vi "Tração cond a AT  subvão.vi"(8 "error in (no error)":errorcluster, 11 "Dados SP":T1={"Condutor"={"Pc (N/m)"=0.0, "Mod.Young (N/m²)"=0.0, "Dil.Term.c (m/°C)"=0.0, "Área  (m²)"=0.0, "Tração EDS (N)"=0.0, "Tração Torig(N)"=0.0, "Tração Talta (N)"=0.0}, "Suporte"={"Ps (N/m)"=0.0, "Es (N/m²)"=0.0, "DTc (1/°C)"=0.0, "Área sup (m²)"=0.0, "Tração EDS sup (N)"=0.0, "Tração AT sup (N)"=0.0, "Flecha sup AT (m)"=0.0}, "Projeto"={"Temp. EDS (°C)"=0.0, "Lim.original (°C)"=0.0, "Lim.extend. (°C)"=0.0, "N. cabo/fase"=1.0}, "Vetor de dados"={"Coor.X.esp"=[], "Coor.Y.Esp."=[], "Sub.vao X"=[], "Sub.vao Y"=[], "CoordY.sup"=[], "CoordX.sup"=[]}, "Subvão"={"N. Esp."=0.0, "F.lim (m)"=0.0, "Ext.calc"=0.0, "Ext.definido"=0.0, "Comp.cabo"=0.0, "Ext.55%"=0.0, "Tração sub\nAT (N)"=0.0, "Ext.sel."=0.0, "Flecha lim.\ncalc (m)"=0.0}, "Vão"={"Extensão (m)"=0.0, "Desnivel (m)"=0.0, "Ext.Lim sub (m)"=0.0, "Flecha à 60 °C"=0.0}} {"Projeto"."N. cabo/fase" min=1.0 max=8.0 step=1.0 format="%#_1f"}) -> (0 "error out":errorcluster, 3 "Dados SP Out":T1={"Condutor"={"Pc (N/m)"=0.0, "Mod.Young (N/m²)"=0.0, "Dil.Term.c (m/°C)"=0.0, "Área  (m²)"=0.0, "Tração EDS (N)"=0.0, "Tração Torig(N)"=0.0, "Tração Talta (N)"=0.0}, "Suporte"={"Ps (N/m)"=0.0, "Es (N/m²)"=0.0, "DTc (1/°C)"=0.0, "Área sup (m²)"=0.0, "Tração EDS sup (N)"=0.0, "Tração AT sup (N)"=0.0, "Flecha sup AT (m)"=0.0}, "Projeto"={"Temp. EDS (°C)"=0.0, "Lim.original (°C)"=0.0, "Lim.extend. (°C)"=0.0, "N. cabo/fase"=1.0}, "Vetor de dados"={"Coor.X.esp"=[], "Coor.Y.Esp."=[], "Sub.vao X"=[], "Sub.vao Y"=[], "CoordY.sup"=[], "CoordX.sup"=[]}, "Subvão"={"N. Esp."=0.0, "F.lim (m)"=0.0, "Ext.calc"=0.0, "Ext.definido"=0.0, "Comp.cabo"=0.0, "Ext.55%"=0.0, "Tração sub\nAT (N)"=0.0, "Ext.sel."=0.0, "Flecha lim.\ncalc (m)"=0.0}, "Vão"={"Extensão (m)"=0.0, "Desnivel (m)"=0.0, "Ext.Lim sub (m)"=0.0, "Flecha à 60 °C"=0.0}} {"Projeto"."N. cabo/fase" min=1.0 max=8.0 step=1.0 format="%#_1f"})   [LabVIEW 2020]
uses:
  controles/SP data.ctl
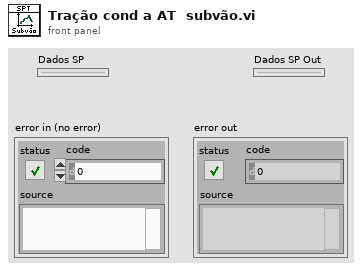
[diagram p1: front panel]
types:
  T1 = typedef "SP data.ctl" = cluster{"Condutor":cluster{"Pc (N/m)":dbl, "Mod.Young (N/m²)":dbl, "Dil.Term.c (m/°C)":dbl, "Área  (m²)":dbl, "Tração EDS (N)":dbl, "Tração Torig(N)":dbl, "Tração Talta (N)":dbl}, "Suporte":cluster{"Ps (N/m)":dbl, "Es (N/m²)":dbl, "DTc (1/°C)":dbl, "Área sup (m²)":dbl, "Tração EDS sup (N)":dbl, "Tração AT sup (N)":dbl, "Flecha sup AT (m)":dbl}, "Projeto":cluster{"Temp. EDS (°C)":dbl, "Lim.original (°C)":dbl, "Lim.extend. (°C)":dbl, "N. cabo/fase":dbl}, "Vetor de dados":cluster{"Coor.X.esp":dbl[], "Coor.Y.Esp.":dbl[], "Sub.vao X":dbl[], "Sub.vao Y":dbl[], "CoordY.sup":dbl[], "CoordX.sup":dbl[]}, "Subvão":cluster{"N. Esp.":dbl, "F.lim (m)":dbl, "Ext.calc":dbl, "Ext.definido":dbl, "Comp.cabo":dbl, "Ext.55%":dbl, "Tração sub\nAT (N)":dbl, "Ext.sel.":dbl, "Flecha lim.\ncalc (m)":dbl}, "Vão":cluster{"Extensão (m)":dbl, "Desnivel (m)":dbl, "Ext.Lim sub (m)":dbl, "Flecha à 60 °C":dbl}}
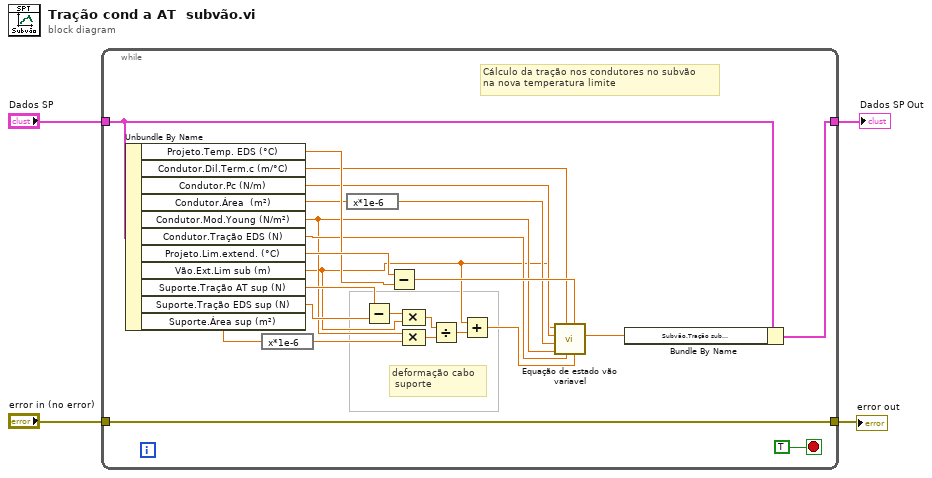
[diagram p0: block diagram]
diagram:
  n1 = while {
    tunnel: "Dados SP" -> [w26]
    tunnel: [w25] -> w3
    tunnel: [w28] -> w1
    tunnel: "error in (no error)" -> [w28]
    stop <- TRUE stop-if-true
    # "deformação cabo\n suporte"
    # "Cálculo da tração nos condutores no subvão\nna nova temperatura limite"
    n2 = Unbundle By Name(w26) -> ("Projeto.Temp. EDS (°C)"=w23:dbl, "Condutor.Dil.Term.c (m/°C)"=w21:dbl, "Condutor.Pc (N/m)"=w20:dbl, "Condutor.Área  (m²)"=w19:dbl, "Condutor.Mod.Young (N/m²)"=w10:dbl, "Condutor.Tração EDS (N)"=w18:dbl, "Projeto.Lim.extend. (°C)"=w24:dbl, "Vão.Ext.Lim sub (m)"=w5:dbl, "Suporte.Tração AT sup (N)"=w13:dbl, "Suporte.Tração EDS sup (N)"=w12:dbl, "Suporte.Área sup (m²)"=w8:dbl)
    n3 = expression code="x*1e-6"(w8) -> (w7:dbl)
    n4 = expression code="x*1e-6"(w19) -> (w9:dbl)
    n5 = Subtract(x=w13, y=w12) -> (x-y=w11:dbl)
    n6 = Subtract(x=w24, y=w23) -> (x-y=w22:dbl)
    n7 = Compound Arithmetic op=MULTIPLY(w11, w5) -> (w14:dbl)
    n8 = Compound Arithmetic op=MULTIPLY(w10, w7) -> (w15:dbl)
    n9 = Divide(x=w14, y=w15) -> (x/y=w16:dbl)
    n10 = Add(x=w5, y=w16) -> (x+y=w6:dbl)
    n11 = call "Equação de estado vão variavel.vi"("A1 (m)"=w6, "t2-t1 (°C)"=w22, "To1 (N)"=w18, "Alfa t (1/°C)"=w21, "E (Pa)"=w10, "S (m²)"=w9, "p (N/m)"=w20, "Ao (m)"=w5) -> ("To2 Real  (N)"=w17:dbl)  [unwired: 3 in]
    n12 = Bundle By Name(cluster=w26, "Subvão.Tração sub\nAT (N)"=w17) -> (w25:T1)
  }
  "Dados SP Out" <- w3
  "error out" <- w1
